vi "Build VGA buffer.vi"() -> ()   [LabVIEW 2015]
panel:
  out "VGA data 2":i16[](array[numeric])=[15000, 15000, 15000, 15000, 15000, 15000, 15000, 15000, 15000, 15000, 15000, 15000, 15000, 15000, 15000, 15000, 15000, 15000, 15000, 15000, 15000, 15000, 15000, 15000, 15000, 15000, 15000, 15000, 15000, 15000, 15000, 15000, 15000, 15000, 15000, 15000, 15000, 15000, 15000, 15000, 15000, 15000, 15000, 15000, 15000, 15000, 15000, 15000, 15000, 15000, 15000, 15000, 15000, 15000, 15000, 15000, 15000, 15000, 15000, 15000, 15000, 15000, 15000, 15000, 15000, 15000, 15000, 15000, 15000, 15000, 15000, 15000, 15000, 15000, 15000, 15000, 15000, 15000, 15000, 15000, 15000, 15000, 15000, 15000, 15000, 15000, 15000, 15000, 15000, 15000, 15000, 15000, 15000, 15000, 15000, 15000, 15000, 15000, 15000, 15000]
  out "Array":u8[](array[numeric])
  out "VGA data":i16[](array[numeric])
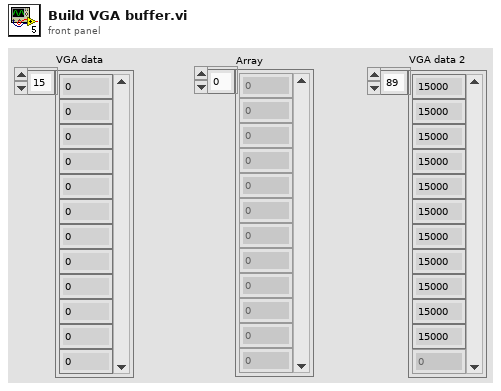
[diagram p1: front panel]
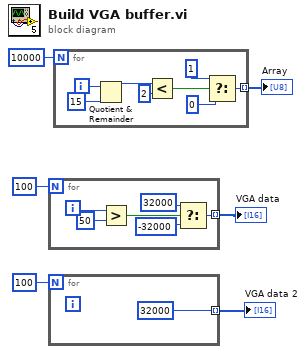
[diagram p0: block diagram]
diagram:
  n1 = for {
    N: 100 -> [_]
    tunnel: [w7] -> w4 mode=indexing
    i -> [w12]
    n2 = Greater?(x=w12, y=50) -> (0:w10:bool)
    n3 = Select(t=32000, s=w10, f=-32000) -> (s? t:f=w7:i32)
  }
  "VGA data" <- w4
  n4 = for {
    N: 100 -> [_]
    tunnel: [32000] -> w1 mode=indexing
  }
  "VGA data 2" <- w1
  n5 = for {
    N: 10000 -> [_]
    tunnel: [w17] -> w3 mode=indexing
    i -> [w21]
    n6 = Quotient & Remainder(x=w21, y=15) -> (x-y*floor(x/y)=w16:i32)  [unwired: 1 out]
    n7 = Less?(x=w16, y=2) -> (x < y?=w14:bool)
    n8 = Select(t=u8 1, s=w14, f=u8 0) -> (s? t:f=w17:u8)
  }
  "Array" <- w3
